vi "Reset.vi"(8 "error in (no error)":errorcluster, 11 "VISA resource name":refnum<visa-resource-name>) -> (0 "error out":errorcluster, 3 "VISA resource name out":refnum<visa-resource-name>)   [LabVIEW 2014, in "Associated Research SC6540.lvlib"]
doc: "Reset the instrument by sending *RST command."
uses:
  <instrlib>/Associated Research SC6540/Associated Research SC6540.lvlib
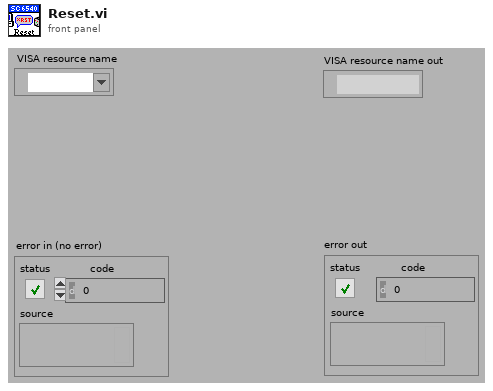
[diagram p1: front panel]
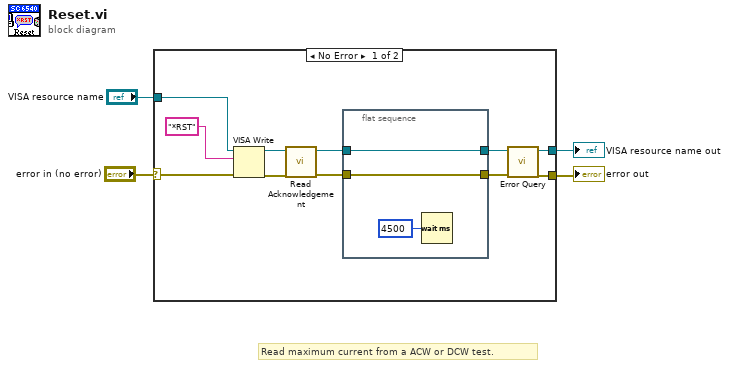
[diagram p0: block diagram]
diagram:
  # "Read maximum current from a ACW or DCW test."
  n1 = case shown="No Error" "error in (no error)" {
    selector: "error in (no error)" -> [w10 w19]
    tunnel: "VISA resource name" -> [w13 w20]
    tunnel: [w12 w20] -> w3
    tunnel: [w11 w19] -> w2
    frame No Error {
      n2 = VISA Write(VISA resource name=w13, write buffer="*RST" ("Command to Send (empty)"), error in (no error)=w10) -> (VISA resource name out=w14:refnum<visa-resource-name>, error out=w15:errorcluster)  [unwired: 1 out]
      n3 = call <instrlib>:"Read Acknowledgement.vi"("error in (no error)"=w15, "VISA resource name"=w14) -> ("error out"=w5:errorcluster, "VISA resource name out"=w8:refnum<visa-resource-name>)  [unwired: 8 in]
      n4 = flat-sequence {
        tunnel: w8 -> [w18]
        tunnel: [w18] -> w7
        tunnel: [w17] -> w6
        tunnel: w5 -> [w17]
        frame #0 {
          n5 = Wait (ms)(milliseconds to wait=u32 4500) -> ()  [unwired: 1 out]
        }
      }
      n6 = call <instrlib>:"Error Query.vi"("error in (no error)"=w6, "VISA resource name"=w7) -> ("error out"=w11:errorcluster, "VISA resource name out"=w12:refnum<visa-resource-name>)  [unwired: 6 in, 2 out]
    }
    frame Error {
    }
  }
  "error out" <- w2
  "VISA resource name out" <- w3
